vi "OE2052_Data Index.vi"(1 "Parameter Type":u16(ring) items=["A_X", "A_Y", "A_R", "A_θ", "A_Frequency", "B_X", "B_Y", "B_R", "B_θ", "B_Frequency"], 2 "Input Date Array":dbl[](array[numeric])) -> (0 "Parameter":dbl)   [LabVIEW 2011]
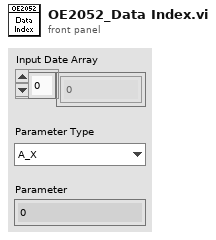
[diagram p1: front panel]
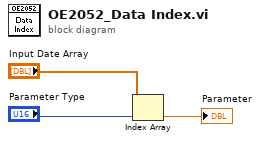
[diagram p0: block diagram]
diagram:
  n1 = Index Array(array="Input Date Array", index="Parameter Type") -> (element=→"Parameter":dbl)
